vi "Unit Test.vi"(2 "Wait (ms)":u32=300, 3 "Reads":u8[](array[numeric]), 4 "Commands":u8[](array[numeric])) -> (0 "Readouts":u8[](array[numeric]), 1 "Writes":u8[](array[numeric]))   [LabVIEW 2018]
uses:
  <vilib>/rvi/interface/RandomDataEmulation/nirviRandomDataOpen.vi
  <vilib>/rvi/interface/common/niFpgaCacheSessionInfoDynamic.vi
  <vilib>/FPGAPlugInAG/Dynamic/niLvFpga_Run_Dynamic.vi
  <vilib>/Utility/error.llb/Error Cluster From Error Code.vi
  <vilib>/rvi/errors/niLvFpgaAdjustHostInterfaceError.vi
  <vilib>/FPGAPlugInAG/Dynamic/niLvFpga_Close_Dynamic.vi
  <vilib>/rvi/interface/nirviOpenFPGA/nirviOpenFPGA.xnode
  FPGATest.vi
  <vilib>/rvi/interface/nirviMethod/nirviMethod.xnode
  <vilib>/rvi/interface/nirviCloseFPGA/nirviCloseFPGA.xnode
  <vilib>/rvi/errors/niLvFpgaMergeErrorWithErrorCode.vi
  <vilib>/FPGAPlugInAG/Dynamic/niLvFpga_WriteFifo_Dynamic.vi
  <vilib>/FPGAPlugInAG/Dynamic/niLvFpga_ReadFifo_Dynamic.vi
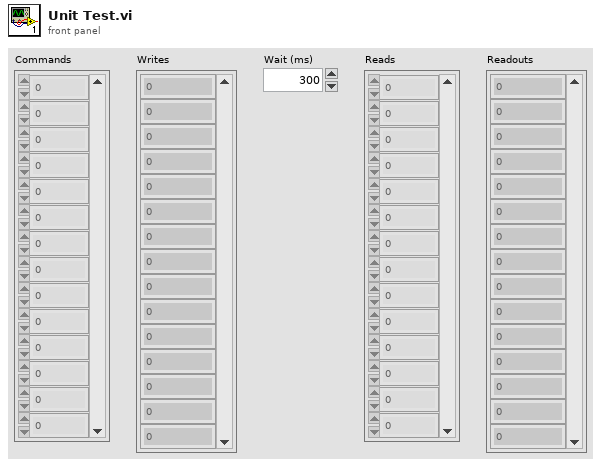
[diagram p1: front panel]
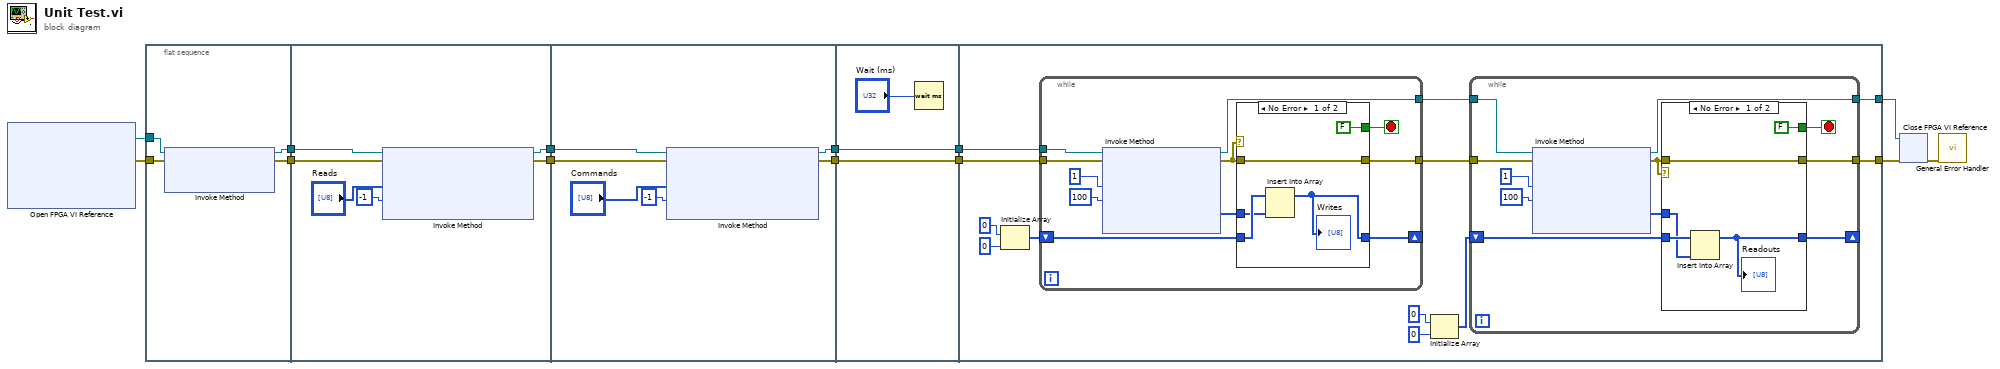
[diagram p0: block diagram]
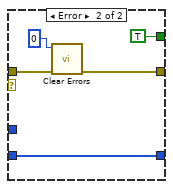
[diagram p2: hidden frame]
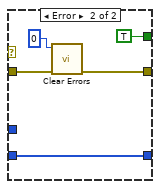
[diagram p3: hidden frame]
diagram:
  n1 = xnode "Open FPGA VI Reference"() -> ("FPGA VI Reference Out"=w11:refnum<k20>, "error out"=w10:errorcluster)  [unwired: 2 in]
  n2 = flat-sequence {
    tunnel: w10 -> [w16]
    tunnel: w11 -> [w17]
    tunnel: [w15] -> w13
    tunnel: [w14] -> w12
    tunnel: w13 -> [w18]
    tunnel: w12 -> [w19]
    tunnel: [w21] -> w7
    tunnel: [w20] -> w6
    tunnel: [w24] -> w5
    tunnel: [w25] -> w3
    tunnel: w7 -> [w27]
    tunnel: w6 -> [w26]
    tunnel: w5 -> [w32]
    tunnel: [w32] -> w4
    tunnel: w3 -> [w31]
    tunnel: [w31] -> w2
    tunnel: [w34] -> w8
    tunnel: w4 -> [w44]
    tunnel: w2 -> [w43]
    tunnel: [w33] -> w9
    frame #0 {
      n3 = xnode "Invoke Method"("FPGA VI Reference In"=w17, "error in"=w16) -> ("FPGA VI Reference Out"=w14:refnum<k20>, "error out"=w15:errorcluster)  [unwired: 1 in]
    }
    frame #1 {
      n4 = xnode "Invoke Method"("FPGA VI Reference In"=w19, "error in"=w18, "Data"="Reads", "Timeout (ms)"=-1) -> ("FPGA VI Reference Out"=w21:refnum<k20>, "error out"=w20:errorcluster)  [unwired: 1 out]
    }
    frame #2 {
      n5 = xnode "Invoke Method"("FPGA VI Reference In"=w27, "error in"=w26, "Data"="Commands", "Timeout (ms)"=-1) -> ("FPGA VI Reference Out"=w24:refnum<k20>, "error out"=w25:errorcluster)  [unwired: 1 out]
    }
    frame #3 {
      n6 = Wait (ms)(milliseconds to wait="Wait (ms)") -> ()  [unwired: 1 out]
    }
    frame #4 {
      n7 = Initialize Array(u8 0 ("element"), 0 ("dimension size")) -> (w40:u8[])
      n8 = while {
        tunnel: w44 -> [w73]
        tunnel: w43 -> [w74]
        tunnel: [w70] -> w35
        shift-right: [w69] -> _
        shift-left: w40 -> [w72]
        tunnel: [w68] -> w36
        stop <- w67 stop-if-true
        n9 = xnode "Invoke Method"("FPGA VI Reference In"=w73, "error in"=w74, "Number of Elements"=u32 1, "Timeout (ms)"=100) -> ("FPGA VI Reference Out"=w68:refnum<k20>, "error out"=w66:errorcluster, "Data"=w71:u8[])  [unwired: 1 out]
        n10 = case shown="No Error" w66 {
          tunnel: w72 -> [w81 w86]
          tunnel: w71 -> [w80 _]
          tunnel: [w79 w86] -> w69
          tunnel: [w78 w82] -> w70
          tunnel: w66 -> [w78 w83]
          tunnel: [FALSE TRUE] -> w67
          frame No Error {
            n11 = Insert Into Array(array=w81, new element=w80) -> (w79:u8[])  [unwired: 1 in]
            "Writes" <- w79
          }
          frame Error {
            n12 = call <vilib>:"Clear Errors.vi"("error in (no error)"=w83, "specific error code to clear (0: all)"=0) -> ("error out"=w82:errorcluster)  [unwired: 4 in, 1 out]
          }
        }
      }
      n13 = Initialize Array(u8 0 ("element"), 0 ("dimension size")) -> (w37:u8[])
      n14 = while {
        tunnel: w36 -> [w52]
        tunnel: w35 -> [w53]
        tunnel: [w49] -> w34
        shift-right: [w48] -> _
        shift-left: w37 -> [w51]
        tunnel: [w47] -> w33
        stop <- w46 stop-if-true
        n15 = xnode "Invoke Method"("FPGA VI Reference In"=w52, "error in"=w53, "Number of Elements"=u32 1, "Timeout (ms)"=100) -> ("FPGA VI Reference Out"=w47:refnum<k20>, "error out"=w45:errorcluster, "Data"=w50:u8[])  [unwired: 1 out]
        n16 = case shown="No Error" w45 {
          tunnel: w51 -> [w60 w65]
          tunnel: w50 -> [w59 _]
          tunnel: [w56 w65] -> w48
          tunnel: [w58 w61] -> w49
          tunnel: w45 -> [w58 w62]
          tunnel: [FALSE TRUE] -> w46
          frame No Error {
            n17 = Insert Into Array(array=w60, new element=w59) -> (w56:u8[])  [unwired: 1 in]
            "Readouts" <- w56
          }
          frame Error {
            n18 = call <vilib>:"Clear Errors.vi"("error in (no error)"=w62, "specific error code to clear (0: all)"=0) -> ("error out"=w61:errorcluster)  [unwired: 4 in, 1 out]
          }
        }
      }
    }
  }
  n19 = xnode "Close FPGA VI Reference"("FPGA VI Reference In"=w9, "error in"=w8) -> ("error out"=w1:errorcluster)
  n20 = call <vilib>:"General Error Handler.vi"("error in (no error)"=w1) -> ()  [unwired: 10 in, 5 out]
